vi "LV2G_FilterLookup.vi"(7 "Operation":T1, 8 "error in (no error)":errorcluster, 11 "lookup":string[][](array[string])) -> (0 "error out":errorcluster, 1 "minRange":dbl[](array[numeric]), 2 "maxRange":dbl[](array[numeric]), 3 "lookupOut":string[][](array[string]), 4 "filters":string[](array[string]), 6 "angles":i32[](array[numeric]))   [LabVIEW 2018]
uses:
  <vilib>/Utility/file.llb/Write To Spreadsheet File (string).vi
  <vilib>/Utility/file.llb/Read From Spreadsheet File (string).vi
  Strict Type Controls/Settings Operation.ctl
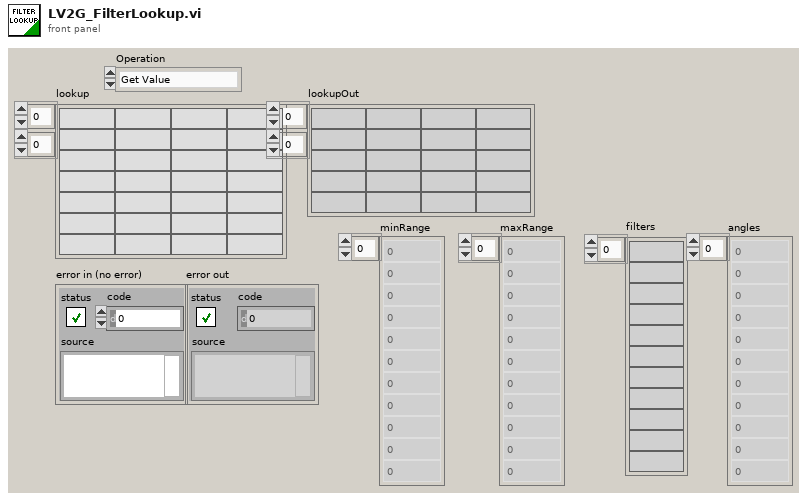
[diagram p1: front panel]
types:
  T1 = typedef "Settings Operation.ctl" = enum8{"Get Value", "Set Value", "Read File", "Write File", "Write Stored Value"}
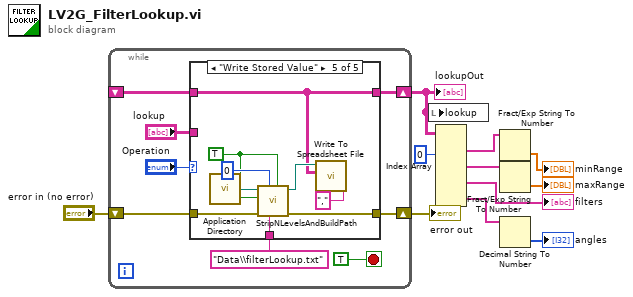
[diagram p0: block diagram]
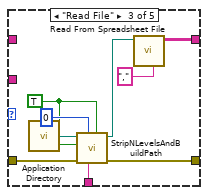
[diagram p4: hidden frame]
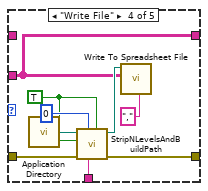
[diagram p5: hidden frame]
diagram:
  n1 = while {
    shift-right: [w18] -> w9
    shift-left: _ -> [w19]
    shift-right: [w15] -> w10
    shift-left: "error in (no error)" -> [w16]
    stop <- TRUE stop-if-true
    n2 = case shown="\"Write Stored Value\"" "Operation" {
      tunnel: w19 -> [w21 _ _ _ w44]
      tunnel: [w21 w23 w26 w35 w44] -> w18
      tunnel: "lookup" -> [_ w23 _ w35 _]
      tunnel: w16 -> [w20 w22 w29 w40 w47]
      tunnel: [w20 w22 w25 w34 w43] -> w15
      tunnel: "Data\\filterLookup.txt" ("Build Path") -> [_ _ w28 w37 w46]
      frame "Get Value" {
      }
      frame "Set Value" {
      }
      frame "Read File" {
        w30 = TRUE ("Is File?")
        n3 = call <vilib>:"Application Directory.vi"() -> ("Application Directory"=w32:path)
        n4 = call "StripNLevelsAndBuildPath.vi"("Create Folders"=w30, "Build Path"=w28, "Strip Levels"=0, "error in(no error)"=w29, "Is File"=w30, "Path In"=w32) -> ("error out"=w25:errorcluster, "Path Out"=w27:path)  [unwired: 4 out]
        n5 = call-poly <vilib>:"Read From Spreadsheet File.vi"("delimiter (\\t)"="," ("delimiter (\\t)"), "file path (dialog if empty)"=w27) -> ("all rows"=w26:string[][])  [unwired: 5 in, 4 out]
      }
      frame "Write File" {
        w38 = TRUE ("Is File?")
        n6 = call <vilib>:"Application Directory.vi"() -> ("Application Directory"=w41:path)
        n7 = call "StripNLevelsAndBuildPath.vi"("Create Folders"=w38, "Build Path"=w37, "Strip Levels"=0, "error in(no error)"=w40, "Is File"=w38, "Path In"=w41) -> ("error out"=w34:errorcluster, "Path Out"=w36:path)  [unwired: 4 out]
        n8 = call-poly <vilib>:"Write To Spreadsheet File.vi"("delimiter (\\t)"="," ("delimiter (\\t)"), "2D data"=w35, "file path (dialog if empty)"=w36) -> ()  [unwired: 5 in, 1 out]
      }
      frame "Write Stored Value" {
        w48 = TRUE ("Is File?")
        n9 = call <vilib>:"Application Directory.vi"() -> ("Application Directory"=w50:path)
        n10 = call "StripNLevelsAndBuildPath.vi"("Create Folders"=w48, "Build Path"=w46, "Strip Levels"=0, "error in(no error)"=w47, "Is File"=w48, "Path In"=w50) -> ("error out"=w43:errorcluster, "Path Out"=w45:path)  [unwired: 4 out]
        n11 = call-poly <vilib>:"Write To Spreadsheet File.vi"("delimiter (\\t)"="," ("delimiter (\\t)"), "2D data"=w44, "file path (dialog if empty)"=w45) -> ()  [unwired: 5 in, 1 out]
      }
    }
  }
  "error out" <- w10
  "lookupOut" <- w9
  n12 = local write "lookup"(w9) -> ()
  n13 = Index Array(array=w9, index (col) #1=0 ("disabled index (col)")) -> (element #1=w7:string[], element #2=w6:string[], element #3=→"filters":string[], element #4=w3:string[])  [unwired: 7 in]
  n14 = Fract/Exp String To Number(string=w7) -> (number=→"minRange":dbl[])  [unwired: 3 in, 1 out]
  n15 = Fract/Exp String To Number(string=w6) -> (number=→"maxRange":dbl[])  [unwired: 3 in, 1 out]
  n16 = Decimal String To Number(string=w3) -> (number=→"angles":i32[])  [unwired: 2 in, 1 out]
